vi "Update Help.vi"(5 "Display State In":T1={"Current Channels Info"=[], "Help Prefix"="", "Max Display Size"=8, "Max Size"=8, "Show Buttons"=TRUE, "Data Valid"=refnum, "Show Range"=FALSE, "Range Items"=[], "Range Index"=[]} caption="State", 7 "Remove Channel":refnum<vi>, 10 "Channel Alias":refnum<vi>, 11 "Channel Name":refnum<vi>) -> ()   [LabVIEW 2021, in "myRIO Channel List.xctl"]
uses:
  <vilib>/myRIO/Common/Express VI Framework/xctls/myRIO Channel List/myRIO Channel List.xctl
  <vilib>/myRIO/Common/Express VI Framework/xctls/myRIO Channel List/State.ctl
  <vilib>/myRIO/Common/Profile Manager Framework/typedefs/Channel Info.ctl
  <vilib>/myRIO/Common/Express VI Framework/typedefs/Data Validate Ref.ctl
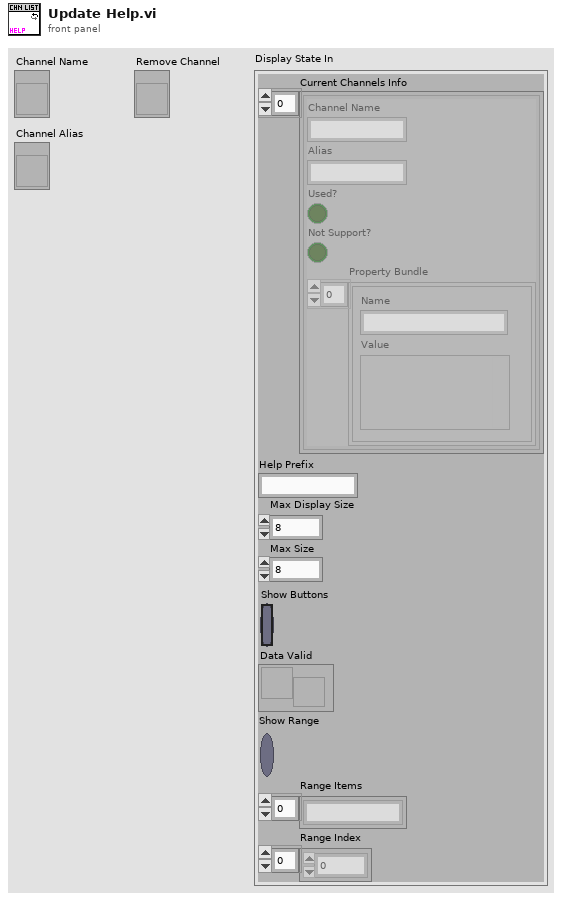
[diagram p1: front panel]
types:
  T1 = typedef "myRIO Channel List.xctl/State.ctl" = cluster{"Current Channels Info":T2[], "Help Prefix":string, "Max Display Size":i32, "Max Size":i32, "Show Buttons":bool, "Data Valid":T3, "Show Range":bool, "Range Items":string[], "Range Index":i32[]}
  T2 = typedef "Channel Info.ctl" = cluster{"Channel Name":string, "Alias":string, "Used?":bool, "Not Support?":bool, "Property Bundle":cluster{"Name":string, "Value":variant}[]}
  T3 = typedef "Data Validate Ref.ctl" = refnum<user-event>
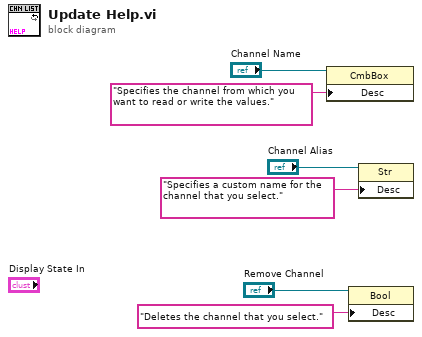
[diagram p0: block diagram]
diagram:
  n1 = property class="CmbBox"(reference="Channel Name", "Desc"="Specifies the channel from which you want to read or write the values." ("format string")) -> ()  [unwired: 1 in, 2 out]
  n2 = property class="Bool"(reference="Remove Channel", "Desc"="Deletes the channel that you select." ("format string")) -> ()  [unwired: 1 in, 2 out]
  n3 = property class="Str"(reference="Channel Alias", "Desc"="Specifies a custom name for the channel that you select." ("format string")) -> ()  [unwired: 1 in, 2 out]
